vi "Repeating Error Handler.vi"   [LabVIEW 2017]
doc: "This merge VI includes additional structures needed to enable the \"retry\" option of the Specific Error Handler. See the Specific Error Handler VI for more information."
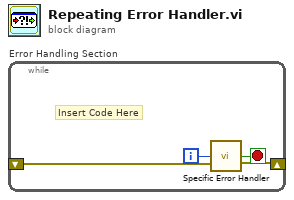
[diagram p0: block diagram]
diagram:
  n1 = while "Error Handling Section" {
    shift-right: [w2] -> _
    shift-left: _ -> [w4]
    i -> [w3]
    stop <- w1 stop-if-true
    # "Insert Code Here"
    n2 = call "Specific Error Handler"("Iteration"=w3, "Error to Check"=w4) -> ("Loop?"=w1:bool, "error out"=w2:errorcluster)  [unwired: 10 in, 2 out]
  }
